vi "init_DAQ.vi"(9 "Sample rate":dbl=100000.0, 10 "Slow/Zelux frame frequency":dbl=20.0, 11 "Fast/Kinetix frame frequency":dbl=100.0) -> (0 "error out":errorcluster, 1 "shutter trigger task":refnum<k21>, 2 "Kinetix trigger task":refnum<k21>, 3 "galvo driving task":refnum<k21>, 4 "Zelux timing read task":refnum<k21>, 5 "Kinetix timing read task":refnum<k21>, 6 "Zelux trigger task":refnum<k21>)   [LabVIEW 2025]
uses:
  <vilib>/DAQmx/create/channels.llb/DAQmx Create Channel (AO-Voltage-Basic).vi
  <vilib>/DAQmx/create/channels.llb/DAQmx Create Channel (CO-Pulse Generation-Frequency).vi
  <vilib>/DAQmx/create/channels.llb/DAQmx Create Channel (AI-Voltage-Basic).vi
  <vilib>/DAQmx/configure/timing.llb/DAQmx Timing (Implicit).vi
  <vilib>/DAQmx/configure/timing.llb/DAQmx Timing (Sample Clock).vi
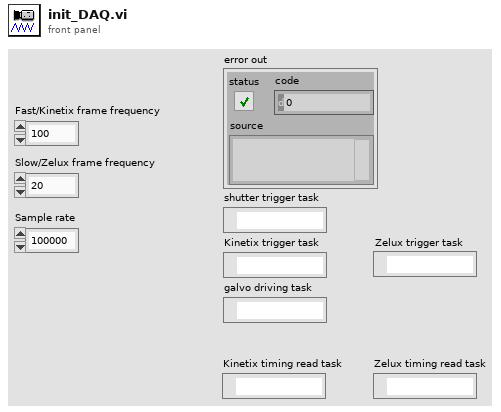
[diagram p1: front panel]
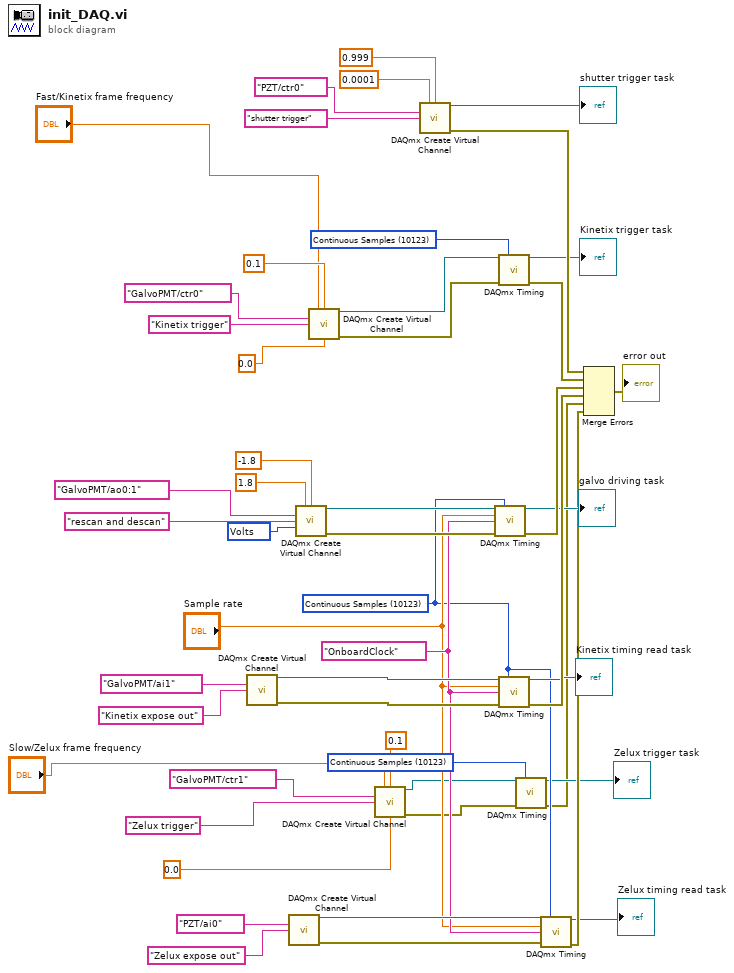
[diagram p0: block diagram]
diagram:
  w5 = 10123 items=["Finite Samples"=10178, "Continuous Samples"=10123, "Hardware Timed Single Point"=12522] ("sample mode")
  w24 = 10123 items=["Finite Samples"=10178, "Continuous Samples"=10123, "Hardware Timed Single Point"=12522] ("sample mode")
  w13 = tag "OnboardClock" ("source")
  w11 = 10123 items=["Finite Samples"=10178, "Continuous Samples"=10123, "Hardware Timed Single Point"=12522] ("sample mode")
  w51 = 10348 items=["Volts"=10348, "From Custom Scale"=10065] ("units")
  n1 = call-poly <vilib>:"DAQmx Create Virtual Channel.vi"("physical channels"=tag "GalvoPMT/ai1", "name to assign"="Kinetix expose out") -> ("task out"=w34:refnum<k21>, "error out"=w35:errorcluster)  [unwired: 12 in]
  n2 = call-poly <vilib>:"DAQmx Create Virtual Channel.vi"("physical channels"=tag "PZT/ai0", "name to assign"="Zelux expose out") -> ("task out"=w14:refnum<k21>, "error out"=w10:errorcluster)  [unwired: 12 in]
  n3 = call-poly <vilib>:"DAQmx Create Virtual Channel.vi"("maximum value"=1.8, "minimum value"=-1.8, "physical channels"=tag "GalvoPMT/ao0:1", "name to assign"="rescan and descan", "units"=w51) -> ("task out"=w39:refnum<k21>, "error out"=w38:errorcluster)  [unwired: 9 in]
  n4 = call-poly <vilib>:"DAQmx Create Virtual Channel.vi"("frequency"="Fast/Kinetix frame frequency", "duty cycle"=0.1, "counter"=tag "GalvoPMT/ctr0", "name to assign"="Kinetix trigger", "initial delay"=0.0) -> ("task out"=w21:refnum<k21>, "error out"=w25:errorcluster)  [unwired: 9 in]
  n5 = call-poly <vilib>:"DAQmx Create Virtual Channel.vi"("frequency"="Slow/Zelux frame frequency", "duty cycle"=0.1, "counter"=tag "GalvoPMT/ctr1", "name to assign"="Zelux trigger", "initial delay"=0.0) -> ("task out"=w3:refnum<k21>, "error out"=w1:errorcluster)  [unwired: 9 in]
  n6 = call-poly <vilib>:"DAQmx Create Virtual Channel.vi"("frequency"=0.0001, "duty cycle"=0.999, "counter"=tag "PZT/ctr0", "name to assign"="shutter trigger") -> ("task out"=→"shutter trigger task":refnum<k21>, "error out"=w33:errorcluster)  [unwired: 10 in]
  n7 = call-poly <vilib>:"DAQmx Timing.vi"("task/channels in"=w39, "sample mode"=w11, "rate"="Sample rate", "source"=w13, "error in"=w38) -> ("task out"=→"galvo driving task":refnum<k21>, "error out"=w31:errorcluster)  [unwired: 9 in]
  n8 = call-poly <vilib>:"DAQmx Timing.vi"("task/channels in"=w21, "sample mode"=w24, "error in"=w25) -> ("task out"=→"Kinetix trigger task":refnum<k21>, "error out"=w23:errorcluster)  [unwired: 11 in]
  n9 = call-poly <vilib>:"DAQmx Timing.vi"("task/channels in"=w34, "sample mode"=w11, "rate"="Sample rate", "source"=w13, "error in"=w35) -> ("task out"=→"Kinetix timing read task":refnum<k21>, "error out"=w30:errorcluster)  [unwired: 9 in]
  n10 = call-poly <vilib>:"DAQmx Timing.vi"("task/channels in"=w3, "sample mode"=w5, "error in"=w1) -> ("task out"=→"Zelux trigger task":refnum<k21>, "error out"=w2:errorcluster)  [unwired: 11 in]
  n11 = call-poly <vilib>:"DAQmx Timing.vi"("task/channels in"=w14, "sample mode"=w11, "rate"="Sample rate", "source"=w13, "error in"=w10) -> ("task out"=→"Zelux timing read task":refnum<k21>, "error out"=w9:errorcluster)  [unwired: 9 in]
  n12 = Merge Errors(w33, w23, w31, w30, w2, w9) -> (→"error out":errorcluster)
